vi "Phoenix.vi"(11 "Args":string[](array[string])) -> (2 "Logs":string, 3 "Exit":i32)   [LabVIEW 2020]
uses:
  Vision_class/Old vision/Controls/Estimadores.ctl
  Vision_class/Old vision/Decode SSL and Refree Wrapper Package Folder/SSL Referee Game Status.ctl
  Vision_class/Old vision/Draw Field Folder/DrawTargets.ctl
  Vision_class/Old vision/Controls/SSL Field State.ctl
  Vision_class/Old vision/Controls/SSL Detection Frame.ctl
  Vision_class/Old vision/Controls/SSL Detection Robot.ctl
  <vilib>/Analysis/Matrix/Datatypes/RealMatrix.ctl
  Vision_class/Old vision/Controls/SSL Detection Ball.ctl
  Communication_class/Communication.lvclass
  Controls/ComUDP.ctl
  Controls/ComSerial.ctl
  Controls/ComSOS.ctl
  Controls/vision_control.ctl
  Team_class/KeeperPlay.ctl
  Team_class/OffensivePlay.ctl
  Referee_class/command_interpreted.ctl
  Robot_class/roles.ctl
  Robot_class/tactics.ctl
  Team_class/DefensivePlay.ctl
  Parameters_class/Project.ctl
  Vision_class/Vision.lvclass
  Game_class/Game.lvclass
  Game_class/Game.lvclass/Game.ctl
  Parameters_class/Parameters.lvclass/Parameters.ctl
  Robot_class/Robot.lvclass
  Team_class/Team.lvclass/Team.ctl
  Events_class/Events.lvclass
  Referee_class/Referee.lvclass/Referee.ctl
  Robot_class/Robot.lvclass/Robot.ctl
  Game_class/Write Offensive ids.vi
  Game_class/Write Defensive ids.vi
  Game_class/Read Parameters.lvclass.vi
  Game_class/Write TestMode IDs.vi
  Game_class/Write TestMode.vi
  Game_class/Write Tests.vi
  Parameters_class/Write Area.vi
  Parameters_class/Write DistanceBehindAttacker.vi
  Parameters_class/Write DistanceInFrontOfAttacker.vi
  Parameters_class/Write DistanceStop.vi
  Parameters_class/Write DistanceToBallOut.vi
  Parameters_class/Write DistanceToGoAroundBall.vi
  Parameters_class/Write DistanceToGoAroundBallPass.vi
  Parameters_class/Write DistanceToKickingAngle.vi
  Parameters_class/Write Force++.vi
  Parameters_class/Write KickAngle.vi
  Parameters_class/Write KickEps.vi
  Parameters_class/Write KickForce.vi
  Parameters_class/Write KickRange.vi
  Parameters_class/Write MaxAcceleration.vi
  Parameters_class/Write MaxControlIncrement.vi
  Parameters_class/Write MaxDeceleration.vi
  Parameters_class/Write MaxOutputAngle.vi
  Parameters_class/Write MaxOutputXY.vi
  Parameters_class/Write MinDistToKick.vi
  Parameters_class/Write PassAngle.vi
  Parameters_class/Write Type of Marker.vi
  Parameters_class/Write AttackerFarback.vi
  Parameters_class/Write TouchDistance.vi
  Parameters_class/Write TimeoutDistanceInY.vi
  Parameters_class/Write TimeoutDistanceInX.vi
  Parameters_class/Write TimeoutDistanceBetweenRobots.vi
  Parameters_class/Write DistanceForPossession.vi
  Parameters_class/Write DistanceForaStillBall.vi
  Parameters_class/Write AngularToleranceForPossession.vi
  Parameters_class/Write AttakingOurselves.vi
  Parameters_class/Write Debug.vi
  Parameters_class/Write ChipKick activated.vi
  Parameters_class/Write Angle.vi
  Parameters_class/Write PID gains Vel.vi
  Parameters_class/Write PID gains Vel_desired.vi
  Parameters_class/Write PID gains Angle.vi
  Parameters_class/Write Number of Offesnive.vi
  Parameters_class/Write Shoot Out_.vi
  Parameters_class/Write DefenseAvoidArea.vi
  Parameters_class/Write InvertKick.vi
  Parameters_class/Write ShootOutForce.vi
  Parameters_class/Write dtPosEstBall.vi
  Parameters_class/Write SimplePass.vi
  Parameters_class/Write GoalieInFrontGoal.vi
  Parameters_class/Write RollToPass.vi
  Parameters_class/Write VelNearBall.vi
  Parameters_class/Write Project.vi
  Game_class/Write Parameters.lvclass.vi
  Game_class/Read DefensiveTeam.vi
  Game_class/Write DefensiveTeam.vi
  Team_class/Read RobotRef.vi
  Game_class/Read OffensiveTeam.vi
  Game_class/Read AllyRef.vi
  Game_class/Read KeeperTeam.vi
  Team_class/Write RobotRef.vi
  Game_class/Write NavigationTeam.vi
  Game_class/Write EventsRef.vi
  Game_class/Write OffensiveTeam.vi
  Game_class/Write KeeperTeam.vi
  Robot_class/Read id.vi
  Robot_class/Read role.vi
  Robot_class/Read tactic.vi
  Game_class/Read Referee.vi
  Team_class/Read DefensivePlay.vi
  Team_class/Read OffensivePlay.vi
  Team_class/Read KeeperPlay.vi
  Referee_class/Read command_interpreted.vi
  Ally_class/Ally.lvclass
  home/roboime/Documentos/VSS_AI/Team_class/Team.lvclass
  Parameters_class/Parameters.lvclass
  Playbook_class/Playbook.lvclass
  Referee_class/Referee.lvclass
  <vilib>/Analysis/Matrix/NI_Matrix.lvlib
panel:
  out "touch":bool
  in  "Debug":bool
  out "tempo udp":dbl
  in  "ball velocity máx":dbl=20.0
  in  "PID gains Angle":cluster{"(Kc)":dbl, "(Ki)":dbl, "(Kd)":dbl}={"(Kc)"=5.0, "(Ki)"=0.1, "(Kd)"=-1.0}
  in  "PID gains Vel D":cluster{"(Kp)":dbl, "(Ki)":dbl, "(Kd)":dbl}={"(Kp)"=20.0, "(Ki)"=100.0, "(Kd)"=0.5}
  in  "ChipKick activated":bool
  out "error out":errorcluster
  in  "Draw Graphs":bool
  out "zoom":dbl
  in  "Test":bool
  in  "Tab Control":T1(tab)
  in  "SEND?":bool=TRUE
  in  "VSSRef Replacement infos":T2={"Local IP:"="NADA", "Port"=10004, "Server IP:"="192.168.0.100"}
  in  "VSSRef":T3
  in  "Project":T4=enum."VSS"
  in  "Com UDP":T5={"UDP GrSim TX"=TRUE, "Address:"="172.31.17.157", "Port:"=20011}
  in  "Com Serial":T6={"Serial TX"=FALSE, "Porta:"="COM12"}
  in  "Com SOS":T7={"UDP SOS TX "=FALSE, "SOS Port: 2"=10025, "SOS Port: "=10021, "SOS Address:"="192.168.0.101"}
  in  "RefBox UDP RX":T2={"Local IP:"="", "Port"=10003, "Server IP:"="224.5.23.2"}
  out "RefBox RX":bool
  in  "Defense\n stretch":i32=2000
  in  "Defense\n width":i32=1000
  in  "Team":enum16{"Azul", "Amarelo"}(ring) caption="Enum"
  in  "Side":enum16{"Esquerdo", "Direito"}(ring) caption="Enum"
  in  "Goalie":string(combo)="0"
  in  "Command":string(combo)="Auto"
  in  "AttakingOurselves":bool
  out "SSL RX":bool
  in  "SSL UDP RX":T2={"Local IP:"="", "Port"=10002, "Server IP:"="224.0.0.1"}
  in  "FIRASim?":bool=TRUE
  out "KeeperPlay":T8=enum."NormalGame"
  out "OffensivePlay":T9=enum."TestPlay"
  out "Keeper Team":cluster{"id":i32, "role":T10, "tactic":T11}[](array[cluster])
  out "Offensive Team":cluster{"id":i32, "role":T10, "tactic":T11}[](array[cluster])
  out "Defensive Team":cluster{"id":i32, "role":T10, "tactic":T11}[](array[cluster])
  out "DefensivePlay":T12=enum."Halt"
  in  "TestMode IDS":dbl[](array[numeric])
  out "SSL Referee Game Status":T13 {"Time" format="%<%.3X %x>T"; "Blue Timeout Remaining" format="%<%M:%S>t"; "Yellow Timeout Remaining" format="%<%M:%S>t"; "Time Left" format="%<%M:%S>t"}
  out "FPS Offensive":dbl
  out "FPS SetParameters":dbl
  out "FPS Defensive":dbl
  out "FPS Keeper":dbl
  out "FPS Com":dbl
  out "FPS Draw Field":dbl
  out "FPS Graph":dbl
  out "FPS referee":dbl
  out "FPS vision":dbl
  out "FPS Events":dbl
  out "FPS Mouse":dbl
  out "FPS Print Field":dbl
  in  "zigzag Points":cluster{"x":dbl, "y":dbl, "Angle":dbl}[](array[cluster])=[{"x"=-4300.0, "y"=-3000.0, "Angle"=0.0}, {"x"=-4300.0, "y"=3000.0, "Angle"=0.0}, {"x"=-100.0, "y"=3000.0, "Angle"=0.0}, {"x"=-4300.0, "y"=3000.0, "Angle"=0.0}]
  in  "TestMode":bool
  in  "Tests":enum16{"zigzag", "goto"}(ring)
  in  "Offensive ids":dbl[](array[numeric])
  in  "Defensive ids":dbl[](array[numeric])
  out "command_interpreted":T14=enum."Halt"
  out "FPS Navigation":dbl
  out "FPS Read UDP":dbl
  in  "id 3":dbl
  in  "id 2":dbl
  in  "id 1":dbl
  out "Robot":cluster{"Modulo":dbl, "Modulo":dbl}(graph)
  out "Robot":cluster{"Modulo":dbl, "Modulo":dbl}(graph)
  out "Robot":cluster{"Modulo":dbl, "Modulo":dbl}(graph)
  out "ball":dbl(graph)
  in  "Tab Control 2":enum32{"SSL Params", "VSS Params"}(tab)
  in  "AI Parameters":T15={"Defensive Marker"=enum."SecondMostDangerous", "TimeoutDistanceInX"=600.0, "TimeoutDistanceInY"=600.0, "DistanceForStealBall"=0.0, "TouchDist"=130.0, "AttackerFarback"=1500.0, "MinDistToKick"=150.0, "Type of Marker"=enum."BlockEnemyPass", "Type of Defense "=enum."Manmark", "PassAngle"=0.045, "KickRange"=60.0, "KickForce"=100.0, "KickEps"=0.05, "KickAngle"=0.09, "Force++"=15.0, "DistanceToKickingAngle"=150.0, "DistanceToBallOut"=600.0, "DistanceStop"=600.0, "DistanceBehindAttacker"=200.0, "Area"=enum."Square", "DistForPossession"=180.0, "DistanceToGoAroundBallPass"=0.0, "DistanceToGoAroundBall"=200.0, "DistanceInFrontOfAttacker"=200.0, "TimeoutDistanceBetweenRobots"=300.0, "MaxOutputAngle"=4.0, "MaxOutputXY"=1.8, "MaxDeceleration"=1.0, "MaxControlIncrement"=1.0, "MaxAcceleration"=4.0, "AngularToleranceForPossession"=0.3, "MaxVelBallToBeginDuelist"=0.5, "ZigZagAngle"=0.0, "PID gains Vel"={"(Kc)"=0.0, "(Ti, min)"=0.0, "(Td, min)"=0.0}, "Number of Offensive"=enum."Auto", "Shoot Out?"=FALSE, "DefenseAvoidArea"=FALSE, "InvertKick"=[], "shootOutForce "=5.0, "dtPosEst\nBall"=0.3, "AttackerIgnoreBallObstacle"=500.0, "BarrierDistanceToArea"=150.0, "SimplePass"=FALSE, "GoalieInFront\nGoal"=90.0, "RollToPass"=FALSE, "VelNearBall"=0.3, "OldRRT"=FALSE}
  in  "AI Parameters VSS":T16={"Robots ids"={"Goalie"=enum."0", "Attacker"=enum."1", "Defender"=enum."2"}}
  in  "Id camera\ninf dir":dbl=2.0
  in  "Id camera\ninf esq":dbl
  in  "Id camera\nsup dir":dbl=3.0
  in  "Id camera\nsup esq":dbl=1.0
  in  "ignore left?":bool
  in  "ignore rigth?":bool
  in  "Estimador":T17
  in  "Draw Targets?":T18={"Attacker"=TRUE, "Striker"=TRUE, "Goalie"=TRUE, "Defender"=TRUE, "kick"=TRUE, "Est Ball"=TRUE, "Est Robot"=FALSE, "Path S"=FALSE, "Path C"=FALSE, "Dngr.Enemy"=TRUE, "2nd Striker"=TRUE}
  in  "Draw Field":bool=TRUE
  in  "Communication in":refnum<class "Communication.lvclass">
  in  "Frame and Field Size out Ref":T19 {"Detection Frame Out"."robots_blue"."height" format="%+4.3f"; "Detection Frame Out"."robots_blue"."pixel_y" format="%+4.3f"; "Detection Frame Out"."robots_blue"."pixel_x" format="%+4.3f"; "Detection Frame Out"."robots_blue"."orientation" format="%+4.3f"; "Detection Frame Out"."robots_blue"."y" format="%+4.3f"; "Detection Frame Out"."robots_blue"."confidence" format="%4.3f"; "Detection Frame Out"."robots_blue"."x" format="%+4.3f"; "Detection Frame Out"."robots_yellow"."height" format="%+4.3f"; "Detection Frame Out"."robots_yellow"."pixel_y" format="%+4.3f"; "Detection Frame Out"."robots_yellow"."pixel_x" format="%+4.3f"; "Detection Frame Out"."robots_yellow"."orientation" format="%+4.3f"; "Detection Frame Out"."robots_yellow"."y" format="%+4.3f"; "Detection Frame Out"."robots_yellow"."confidence" format="%4.3f"; "Detection Frame Out"."robots_yellow"."x" format="%+4.3f"}
  out "2D Picture":picture
  in  "SSL Referee Game Status Ref":T13 {"Time" format="%<%.3X %x>T"; "Blue Timeout Remaining" format="%<%M:%S>t"; "Yellow Timeout Remaining" format="%<%M:%S>t"; "Time Left" format="%<%M:%S>t"}
  out "GUI Game Status":T13 {"Time" format="%<%.3X %x>T"; "Blue Timeout Remaining" format="%<%M:%S>t"; "Yellow Timeout Remaining" format="%<%M:%S>t"; "Time Left" format="%<%M:%S>t"}
  # "To execute Test and TestMode(zigzag)\nthe referee command must be Stop"
  # "PID gains vel:\nmakes the estimated velocity\ngoes closer into the desired velocity"
  # "Score"
  # "Red Cards"
  # "Yellow Cards"
  # "Timeouts Left"
  # "Timeout Remaining"
  # "Goalie ID"
  # "left goal"
  # "right goal"
  # "vision computer"
  # "Score"
  # "Red Cards"
  # "Yellow Cards"
  # "Timeouts Left"
  # "Timeout Remaining"
  # "Goalie ID"
  # "Score"
  # "Red Cards"
  # "Yellow Cards"
  # "Timeouts Left"
  # "Timeout Remaining"
  # "Goalie ID"
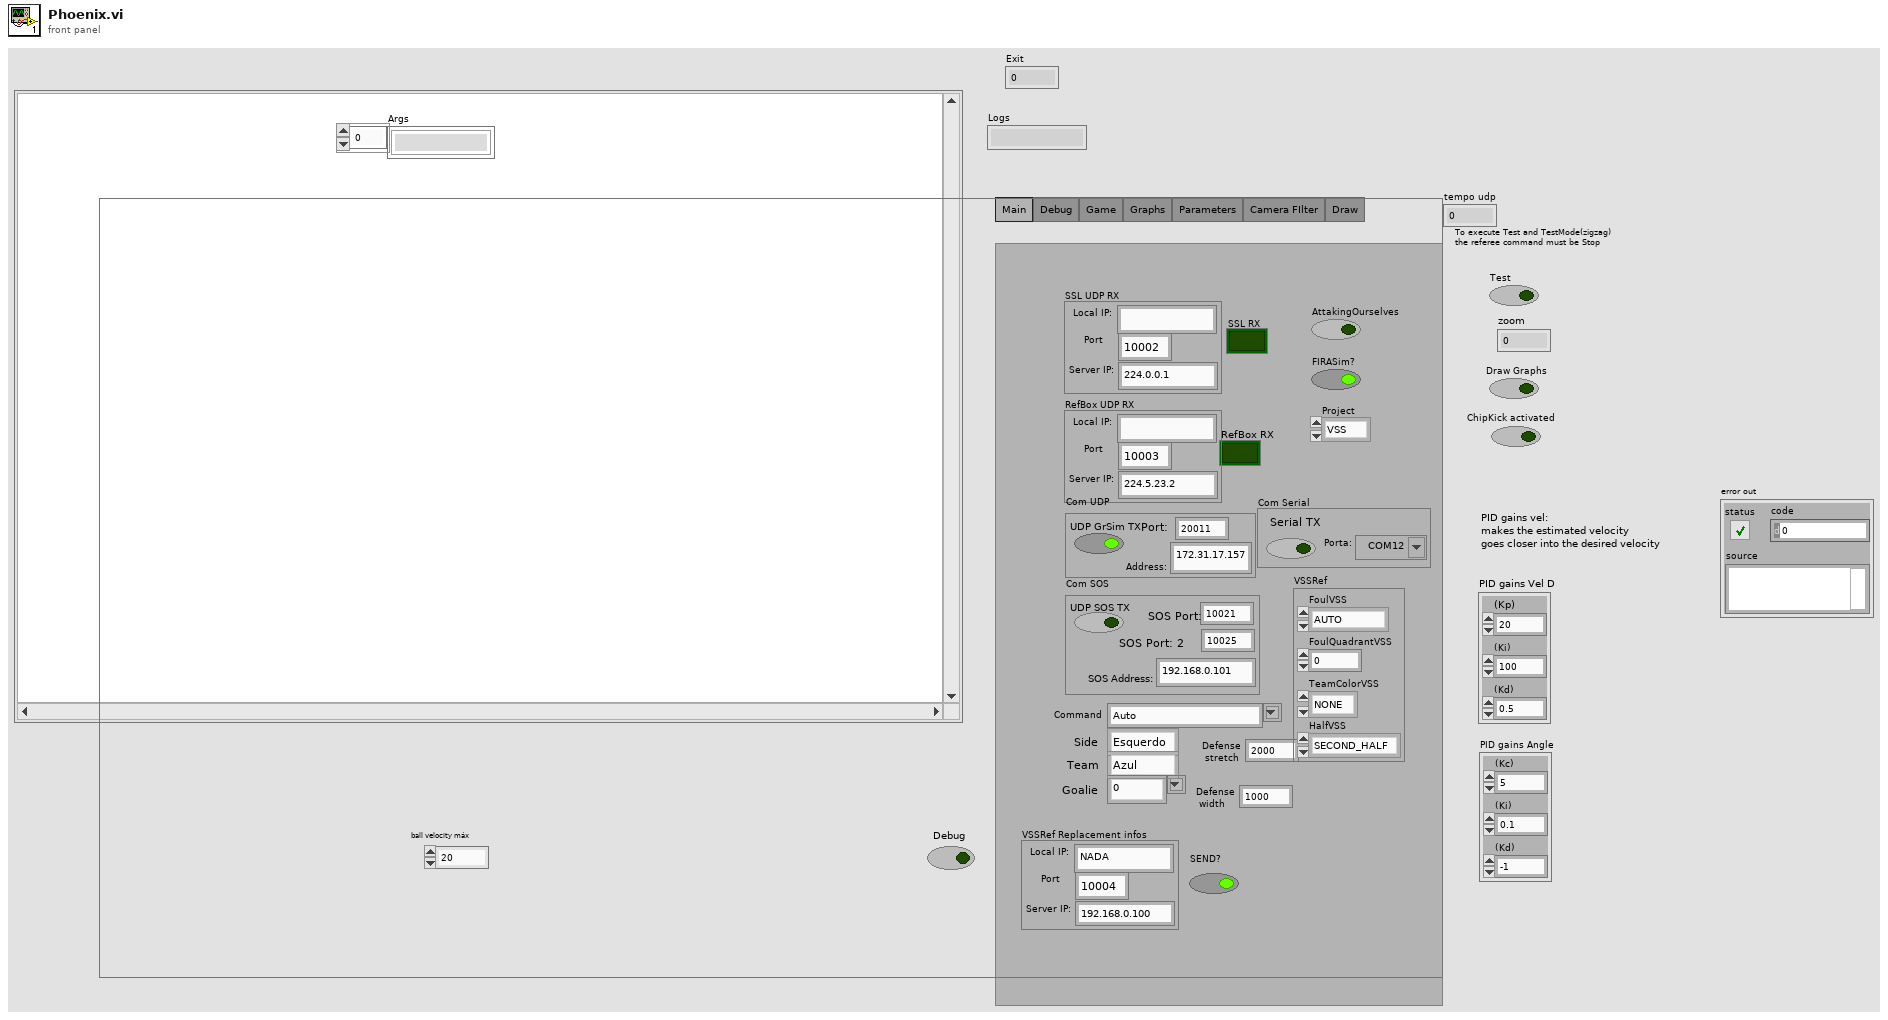
[diagram p1: front panel]
types:
  T1 = enum32{"Main", "Debug", "Game", "Graphs", "Parameters", "Camera FIlter", "Draw"}
  T2 = typedef "vision_control.ctl" = cluster{"Local IP:":string, "Port":i32, "Server IP:":string}
  T3 = cluster{"FoulVSS":enum16{"AUTO", "GAME_ON", "STOP", "KICKOFF", "FREE_BALL", "GOAL_KICK", "PENALTY_KICK", "FREE_KICK"}, "FoulQuadrantVSS":dbl, "TeamColorVSS":enum16{"NONE", "YELLOW", "BLUE"}, "HalfVSS":enum16{"SECOND_HALF", "FIRST_HALF", "NO_HALF"}}
  T4 = typedef "Project.ctl" = enum16{"SSL", "VSS"}
  T5 = typedef "ComUDP.ctl" = cluster{"UDP GrSim TX":bool, "Address:":string, "Port:":u16}
  T6 = typedef "ComSerial.ctl" = cluster{"Serial TX":bool, "Porta:":refnum<visa-resource-name>}
  T7 = typedef "ComSOS.ctl" = cluster{"UDP SOS TX ":bool, "SOS Port: 2":u16, "SOS Port: ":u16, "SOS Address:":string}
  T8 = typedef "KeeperPlay.ctl" = enum16{"ZigZag", "Goto", "NormalGame", "KeeperPlay", "Halt", "Timeout", "PenaltyEnemy", "TestPlay"}
  T9 = typedef "OffensivePlay.ctl" = enum16{"TableWithStriker", "TableWith2ndStrikerPlay", "PrepareDoublePass", "PrepareRollToPass", "SimplePass", "PreparePass", "PassToStriker", "BallOutOfField", "PassTo2ndStriker", "StopOffensive", "Prepare Penalty Enemy", "EnemyPossessionAtEnemyField", "EnemyPossesionAtOurField", "TestPlay", "PreparePenaltyAlly", "KickPenaltyAlly", "PrepareKickoffAlly", "PrepareKickoffEnemy", "IndirectEnemy", "DirectEnemy", "NormalGame", "DirectKick", "Pass", "Halt", "Timeout", "PassPlay", "PenaltyEnemy"}
  T10 = typedef "roles.ctl" = enum16{"BallChallengerAttackerVSS", "NormalAttackerVSS", "AttackerAimGoalVSS", "DefenderAreaVSS", "KeeperVSS", "Tabler", "TableFinalizer", "PrepareRollToPassRoller", "PrepareRollToPassReceiver", "SimplePassRoll", "SimplePassRollReceiver", "PenaltyDefense", "PreparePassReceiver 2", "PreparePassReceiver 1", "PassObserver", "Timeout", "Goto", "ZigZag", "None", "BallOutOfField", "DefenderArea", "Duelist", "AttackerStop", "FollowAttacker", "KeeperRole", "KickPenalty", "AttackerAimGoal", "AttackerBlock", "Marker", "Halt", "Shoot", "PassKicker", "PassReceiver", "TestRole", "PenaltyAttacker"}
  T11 = typedef "tactics.ctl" = enum16{"ReceivePassInFuturePoint", "Roller", "PrepareRollToPassRollerGoTo", "PrepareRollToPassReceiverGoTo", "WaitRoll", "PositionToRoll", "PenaltyAttacker", "PassObserver", "PenaltyDefense", "TableReceiverTactic", "Test", "DefendGoal", "Marker", "FollowAttacker", "DefendArea", "Shoot", "AttackerAimGoal", "AttackerBallOutOfField", "AttackerBlock", "AttackerStop", "Duelist", "Halt", "ZigZag", "GoTo", "Timeout", "KickToPassReceiver", "PositionToReceivePass", "DefendAreaVSS", "DefendGoalVSS", "KickVSS", "AttackVSS", "DispBallVSS", "PenaltyAttackVSS", "WaitPass"}
  T12 = typedef "DefensivePlay.ctl" = enum16{"NormalDefensiveWithDuelist", "NormalDefensive", "TestPlay", "Halt", "Timeout", "PenaltyEnemy", "PenaltyAlly"}
  T13 = typedef "SSL Referee Game Status.ctl" = cluster{"Stage":string, "Command":string, "Time Left":dbl, "Yellow Team":string, "Blue Team":string, "Yellow Score":u32, "Blue Score":u32, "Yellow Red Cards":u32, "Blue Red Cards":u32, "Yellow Yellow Cards":u32, "Blue Yellow Cards":u32, "Yellow Timeouts Left":u32, "Blue Timeouts Left":u32, "Yellow Timeout Remaining":dbl, "Blue Timeout Remaining":dbl, "Yellow Goalie Id":u32, "Blue Goalie Id":u32, "Time":timestamp}
  T14 = typedef "command_interpreted.ctl" = enum16{"Goal Ally", "Goal Enemy", "Ball Placement Enemy", "Ball Placement Ally", "Normal Half Time", "Extra Time  Break", "Extra Half Time", "None", "Post Game", "PKA Normal Start", "Prepare Kickoff Ally", "PKE Normal Start", "Prepare Kickoff Enemy", "Force Start", "Halt", "Timeout", "Prepare Penalty Ally", "Prepare Penalty Enemy", "PPA NormalStart", "PPE Normal Start", "Indirect Free Ally", "Direct Free Enemy", "Direct Free Ally", "Indirect Free Enemy", "Stop"}
  T15 = cluster{"Defensive Marker":enum16{"SecondMostDangerous", "MostDangerous"}, "TimeoutDistanceInX":dbl, "TimeoutDistanceInY":dbl, "DistanceForStealBall":dbl, "TouchDist":dbl, "AttackerFarback":dbl, "MinDistToKick":dbl, "Type of Marker":enum16{"BlockEnemyPass", "BlockOurGoal"}, "Type of Defense ":enum16{"Barreira", "Manmark"}, "PassAngle":dbl, "KickRange":dbl, "KickForce":dbl, "KickEps":dbl, "KickAngle":dbl, "Force++":dbl, "DistanceToKickingAngle":dbl, "DistanceToBallOut":dbl, "DistanceStop":dbl, "DistanceBehindAttacker":dbl, "Area":enum16{"Circular", "Square"}, "DistForPossession":dbl, "DistanceToGoAroundBallPass":dbl, "DistanceToGoAroundBall":dbl, "DistanceInFrontOfAttacker":dbl, "TimeoutDistanceBetweenRobots":dbl, "MaxOutputAngle":dbl, "MaxOutputXY":dbl, "MaxDeceleration":dbl, "MaxControlIncrement":dbl, "MaxAcceleration":dbl, "AngularToleranceForPossession":dbl, "MaxVelBallToBeginDuelist":dbl, "ZigZagAngle":dbl, "PID gains Vel":cluster{"(Kc)":dbl, "(Ti, min)":dbl, "(Td, min)":dbl}, "Number of Offensive":enum16{"6", "5", "4", "3", "2", "1", "0", "Auto"}, "Shoot Out?":bool, "DefenseAvoidArea":bool, "InvertKick":dbl[], "shootOutForce ":dbl, "dtPosEst\nBall":dbl, "AttackerIgnoreBallObstacle":dbl, "BarrierDistanceToArea":dbl, "SimplePass":bool, "GoalieInFront\nGoal":dbl, "RollToPass":bool, "VelNearBall":dbl, "OldRRT":bool}
  T16 = cluster{"Robots ids":cluster{"Goalie":enum16{"auto", "5", "4", "3", "2", "1", "0"}, "Attacker":enum16{"auto", "5", "4", "3", "2", "1", "0"}, "Defender":enum16{"auto", "5", "4", "3", "2", "1", "0"}}}
  T17 = typedef "Estimadores.ctl" = enum16{"4thDerivate", "2ndDerivate", "Nenhum", "Simples", "Kalman"}
  T18 = typedef "DrawTargets.ctl" = cluster{"Attacker":bool, "Striker":bool, "Goalie":bool, "Defender":bool, "kick":bool, "Est Ball":bool, "Est Robot":bool, "Path S":bool, "Path C":bool, "Dngr.Enemy":bool, "2nd Striker":bool}
  T19 = typedef "SSL Field State.ctl" = cluster{"Detection Frame Out":T20, "Field Size Out":cluster{"line_width":u32, "field_length":u32, "field_width":u32, "boundary_width":u32, "referee_width":u32, "goal_width":u32, "goal_depth":u32, "goal_wall_width":u32, "center_circle_radius":u32, "defense_radius":u32, "defense_stretch":u32, "free_kick_from_defense_dist":u32, "penalty_spot_from_field_line_dist":u32, "penalty_line_from_spot_dist":u32}, "Received Time Stamp":timestamp}
  T20 = typedef "SSL Detection Frame.ctl" = cluster{"frame_number":u32, "t_capture":dbl, "t_sent":dbl, "camera_id":u32, "robots_yellow":T21[], "robots_blue":T21[], "balls":T23[], "Valid":bool, "Time Stamp":timestamp, "New":bool, "Initialized":bool}
  T21 = typedef "SSL Detection Robot.ctl" = cluster{"x":sgl, "robot_id":u32, "confidence":sgl, "y":sgl, "orientation":sgl, "pixel_x":sgl, "pixel_y":sgl, "height":sgl, "Valid":bool, "Time Stamp":timestamp, "x_k|k":T22, "Pk|k":T22, "Previous Time Stamp":timestamp, "R":T22, "vx":dbl, "vy":dbl, "vang":dbl}
  T22 = typedef "NI_Matrix.lvlib/RealMatrix.ctl" = dbl[][]
  T23 = typedef "SSL Detection Ball.ctl" = cluster{"x":sgl, "area":u32, "confidence":sgl, "y":sgl, "z":sgl, "pixel_x":sgl, "pixel_y":sgl, "Valid":bool, "Time Stamp":timestamp, "x_k|k":T22, "Pk|k":T22, "Id":u32, "Previous Time Stamp":timestamp, "R":T22, " vx":sgl, "vy":dbl, "vz":dbl}
  T24 = typedef "AI Input.ctl" = cluster{"our_robots":T25[], "enemy_robots":T25[], "balls":T31[], "geometry":T32, "IA Judge":T33, "Received Timestamp":timestamp, "Events":T35}
  T25 = typedef "AI Robot.ctl" = cluster{"id":u32, "function":T26, "x":dbl, "y":dbl, "orientation":dbl, "v_tangent":dbl, "v_normal":dbl, "v_ang":dbl, "kick_x":dbl, "kick_z":dbl, "dribble":bool, "Timestamp":timestamp, "estimatives":cluster{"est_v_tangent":dbl, "est_v_normal":dbl, "est_vx":dbl, "est_vy":dbl, "Pos Robot Est":dbl[]}, "dest_x_kick":dbl, "dest_y_kick":dbl, "Gap Coord":dbl[], "States":T27, "Path ":dbl[][], "Path  Smooth":dbl[][], "Dest":T28, "vx_desired":dbl, "vy_desired":dbl, "slowBehavior":bool, "VSSStates":T30}
  T26 = typedef "Functions Enum.ctl" = enum16{"2nd Striker", "Attacker", "Goalie", "Defender", "Striker", "Goto 0", "Dummy", "Kicker", "ZigZag 0", "ZigZag 1", "ZigZag 2", "ZigZag 3", "ZigZag 4", "ZigZag 5", "ZigZag 6", "ZigZag 7", "ZigZag 8", ""}
  T27 = typedef "AttackerStates.ctl" = enum16{"Pass", "GoToTangent", "BallGetting", "GoToKick", ""}
  T28 = typedef "PathDests.ctl" = T29[]
  T29 = typedef "PathDest.ctl" = cluster{"dest_x":dbl, "dest_y":dbl, "dest_orientation":dbl, "dest_vel":dbl}
  T30 = typedef "VSSAttackerStates.ctl" = enum16{"Pass", "GoToTangent", "BallGetting", "GoToKick", "Rotate anti-clockwise", "Rotate Clockwise", ""}
  T31 = typedef "AI Ball.ctl" = cluster{"x":dbl, "y":dbl, "timestamp":timestamp, "Vel_x":dbl, "Vel_y":dbl, "Pos Bola Est":dbl[], "Valid":bool}
  T32 = typedef "Field Size.ctl" = cluster{"line_width":u32, "field_length":u32, "field_width":u32, "boundary_width":u32, "referee_width":u32, "goal_width":u32, "goal_depth":u32, "goal_wall_width":u32, "center_circle_radius":u32, "defense_radius":u32, "defense_stretch":u32, "free_kick_from_defense_dist":u32, "penalty_spot_from_field_line_dist":u32, "penalty_line_from_spot_dist":u32}
  T33 = typedef "AI Judge.ctl" = cluster{"stage":string, "command":string, "our_goalie_id":dbl, "enemy_goalie_id":dbl, "command enum":T34, "Time":enum16{"Azul", "Amarelo"}}
  T34 = typedef "Command Enum.ctl" = enum16{"Halt", "Stop", "Force Start", "PKA Normal Start", "Prepare Kickoff Ally", "PKE Normal Start", "Prepare Kickoff Enemy", "Prepare Penalty Ally", "PPA Normal Start", "Prepare Penalty Enemy", "PPE Normal Start", "Direct Free Enemy", "Direct Free Ally", "Indirect Free Enemy", "Indirect Free Ally", "Timeout Enemy", "Timeout Ally", "Goal Enemy", "Goal Ally", "Ball Placement Enemy", "Ball Placement Ally", "Normal Half Time", "Extra Time Break", "Extra Half Time", "None", "Post Game"}
  T35 = typedef "Events.ctl" = cluster{"Touch":bool, "Ball out":bool, "id touch":dbl, "Ball out of \nVision":bool, "Ball inside \nGoalie area":bool, "Robot not responding":bool, "Robots responding status":dbl[], "Enemy Ball \nPossession":bool, "Pass State":bool, "id end of pass":dbl, "Kick":bool, "Id ini Possession":dbl, "Ball Possesion":bool, "Id Possesion":dbl, "Direct Kick":bool, "2nd Strk Ativo":bool}
  T36 = cluster{"Varint":u32, "Varint":u32, "Varint":u32, "Double":dbl, "Varint":u32}
  T37 = enum16{"FreeBall", "PrepareFreeBall", "GoalKickEnemy", "GoalKickAlly", "KickoffAlly", "KickoffEnemy", "PrepareGoalKickEnemy", "PrepareGoalKickAlly", "Stop", "PrepareKickoffEnemy", "PrepareKickoffAlly", "PreparePenaltyEnemy", "Timeout", "DeadBall", "NormalGame", "KickPenaltyAlly", "PenaltyEnemy", "BallChallenge", "PreparePenaltyAlly", "Halt"}
  T38 = enum16{"FreeBall", "PrepareFreeBall", "GoalKickEnemy", "GoalKickAlly", "KickoffAlly", "KickoffEnemy", "PrepareGoalKickEnemy", "PrepareGoalKickAlly", "Stop", "PrepareKickoffEnemy", "PrepareKickoffAlly", "PreparePenaltyEnemy", "Timeout", "DeadBall", "NormalGame", "KickPenaltyAlly", "PenaltyEnemy", "BallChallenge", "PreparePenaltyAlly", "Halt"}[]
  T39 = cluster{"(Kc)":dbl, "(Ti, min)":dbl, "(Td, min)":dbl}
  T40 = enum16{"6", "5", "4", "3", "2", "1", "0", "Auto"}
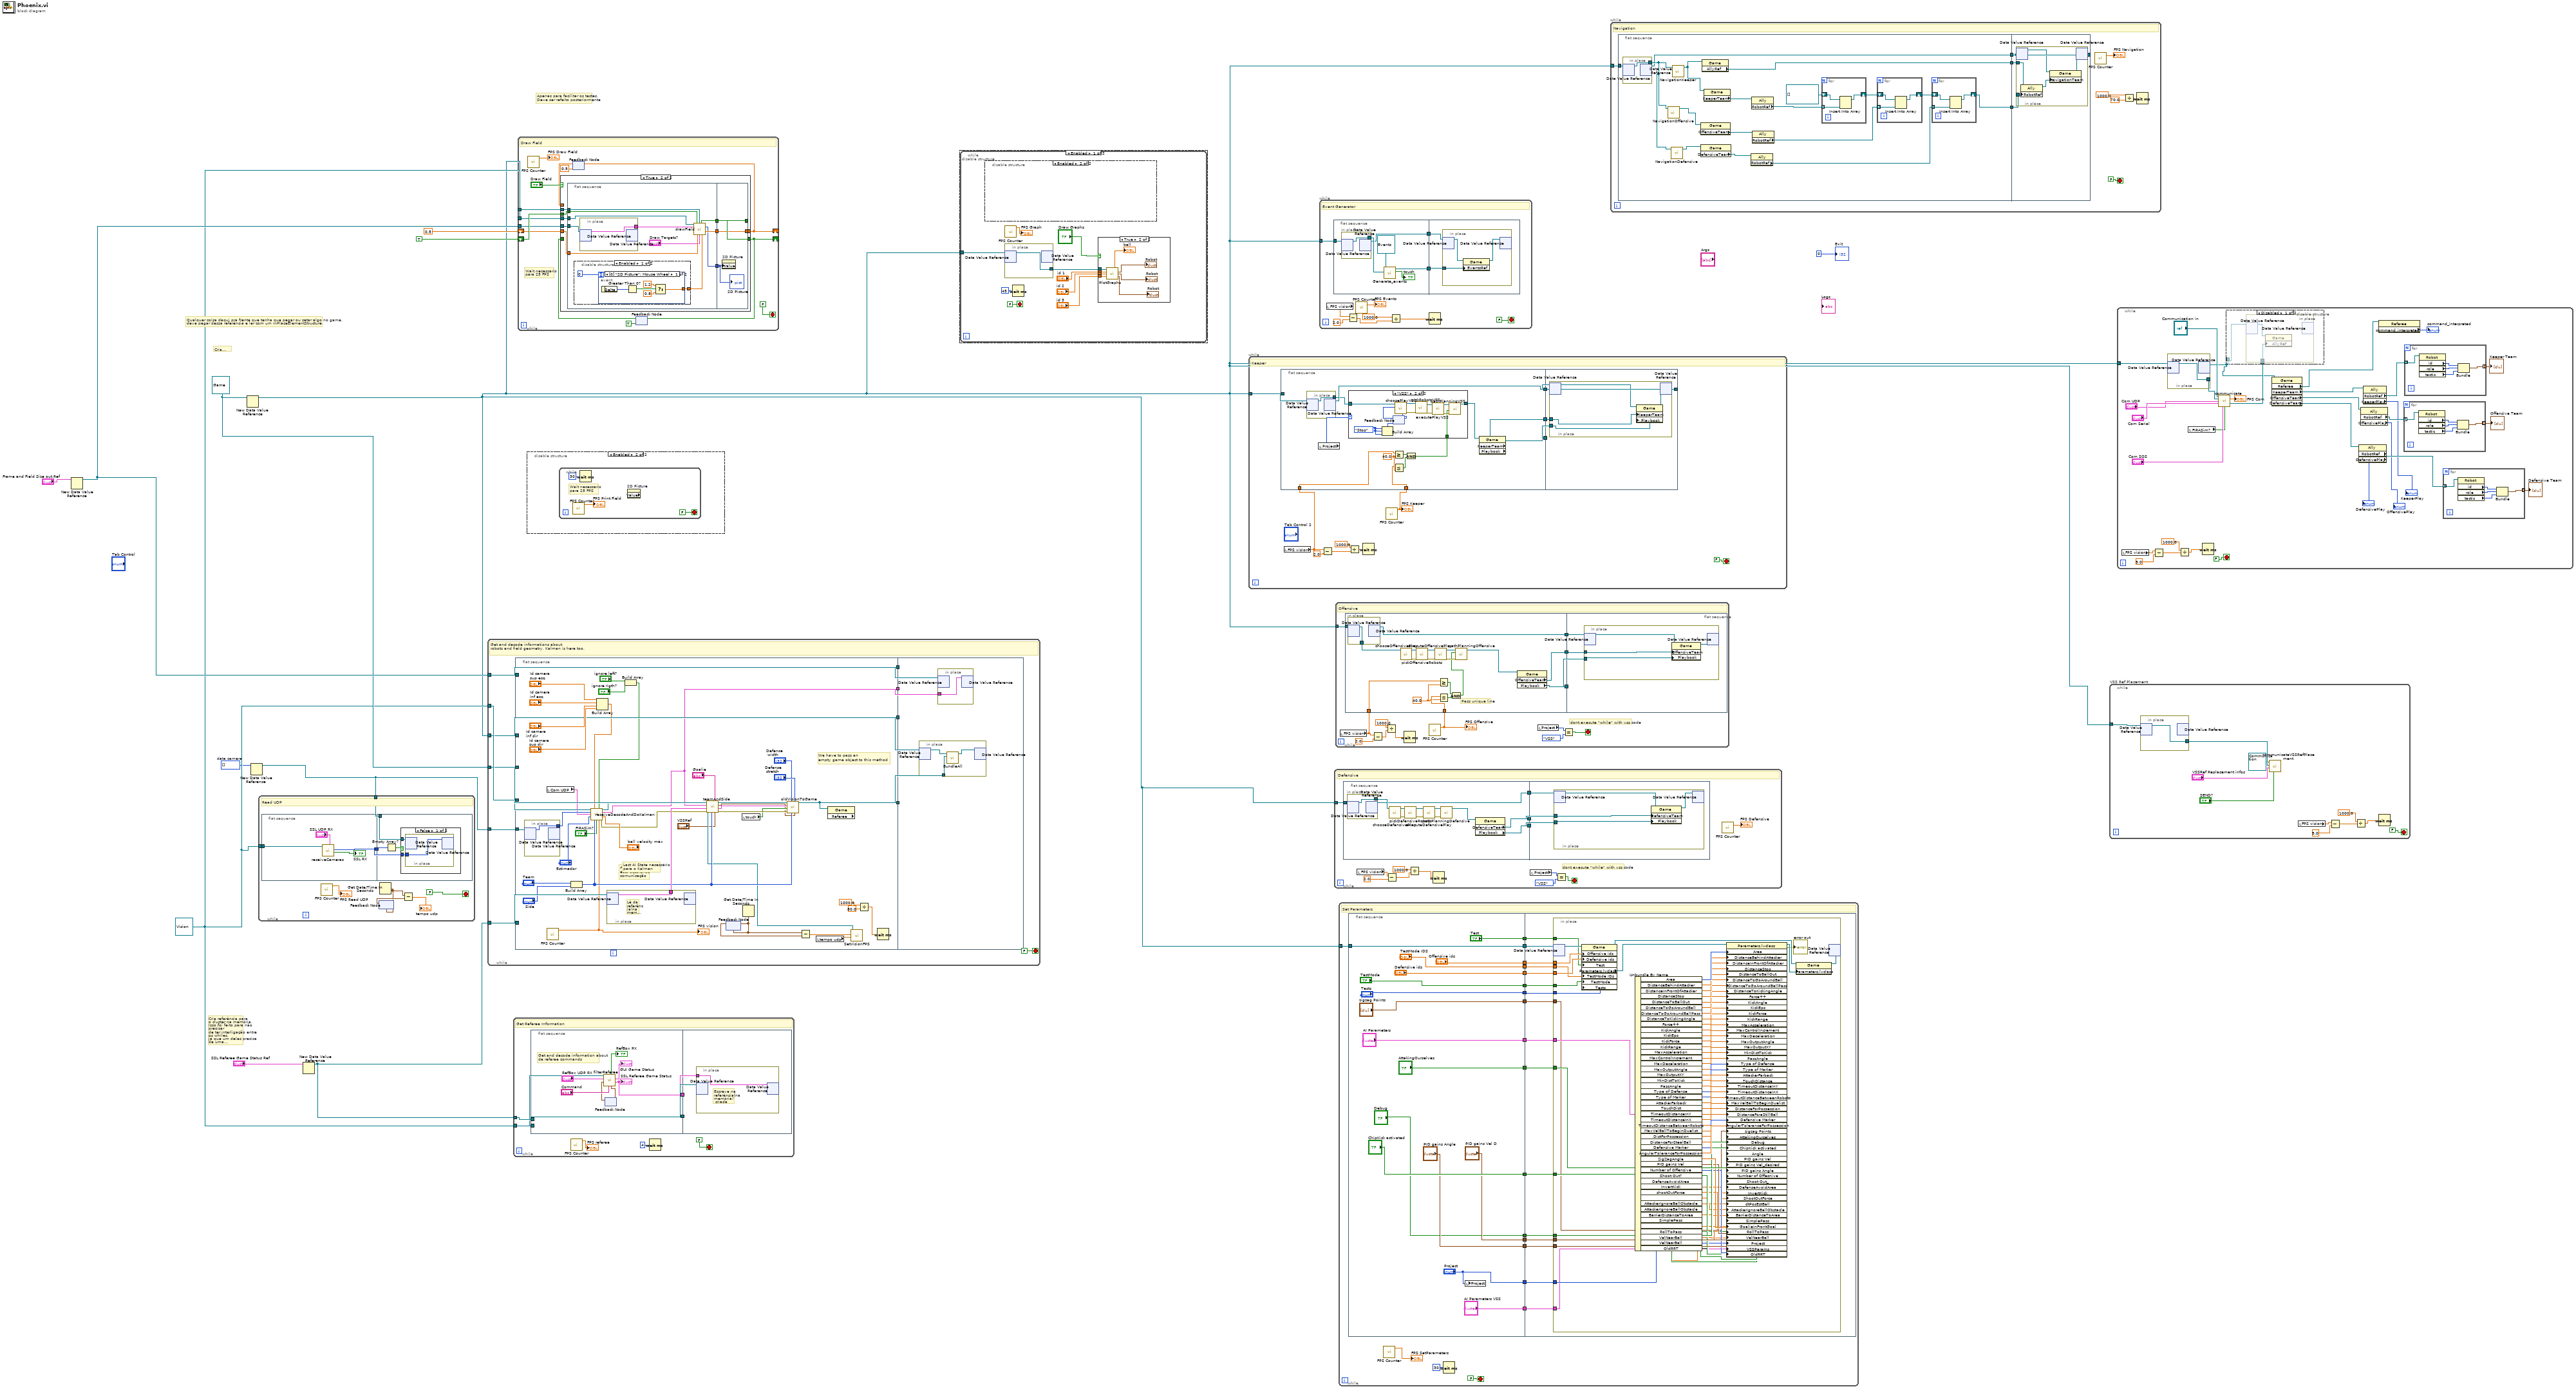
[diagram p0: block diagram]
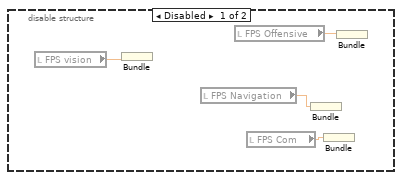
[diagram p3: hidden frame]
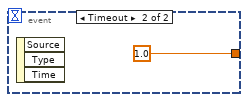
[diagram p7: hidden frame]
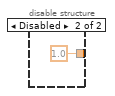
[diagram p8: hidden frame]
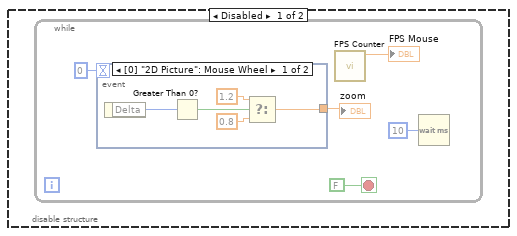
[diagram p9: hidden frame]
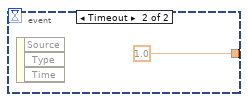
[diagram p10: hidden frame]
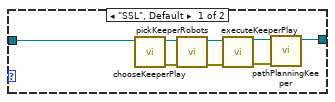
[diagram p11: hidden frame]
diagram:
  w4 = u8[] []  # data camera
  w6 = refnum<class "Game.lvclass"> refnum ("Game")
  w5 = refnum<class "Vision.lvclass"> refnum ("Vision")
  # "Apenas para facilitar os testes.\nDeve ser refeito posteriormente"
  # "Qualquer coisa daqui pra frente que tenha que pegar ou setar algo no game,\ndeve pegar dessa referência e ler com um InPlaceElementStructure"
  # "Cria referência pro game"
  # "Cria referência para\no cluster na memória.\nIsso foi feito para não precisar\nde ter interligação entre os whiles,\njá que um deles precisa de uma\nsaída do outro."
  n1 = New Data Value Reference(data value="Frame and Field Size out Ref") -> (data value reference=w7:refnum<data-value>)  [unwired: 1 in, 1 out]
  n2 = New Data Value Reference(data value=w6) -> (data value reference=w2:refnum<data-value>)  [unwired: 1 in, 1 out]
  n3 = New Data Value Reference(data value=w4) -> (data value reference=w3:refnum<data-value>)  [unwired: 1 in, 1 out]
  n4 = while {
    tunnel: w5 -> [w19]
    tunnel: w3 -> [w18]
    stop <- FALSE stop-if-true
    # "Read UDP"
    n5 = flat-sequence {
      tunnel: w19 -> [w23]
      tunnel: [w22] -> w17
      tunnel: w18 -> [w27]
      tunnel: w17 -> [w26]
      frame #0 {
        n6 = call "receiveCameras.vi"("Cluster"="SSL UDP RX", "Vision in"=w23) -> ("RX"=→"SSL RX":bool, "data camera out"=w22:u8[])  [unwired: 5 in, 2 out]
      }
      frame #1 {
        n7 = Empty Array?(array=w26) -> (empty?=w25:bool)
        n8 = case shown="False" w25 {
          tunnel: w27 -> [w29 _]
          tunnel: w26 -> [w28 _]
          frame False {
            n9 = in-place {
              in-place-border: w28 -> [w30]
              n10 = in-place-dvr #1(w29) -> ()  [unwired: 2 out]
              n11 = in-place-dvr #1(w30) -> ()  [unwired: 2 out]
            }
          }
          frame True {
          }
        }
      }
    }
    n12 = call "FPS Counter.vi"() -> ("Numeric"=→"FPS Read UDP":dbl)  [unwired: 11 in]
    n13 = Get Date/Time In Seconds() -> (seconds since 1Jan1904=w14:timestamp)
    n14 = feedback #2(w14) -> (w15:timestamp)
    n15 = feedback-in #2(w14) -> ()
    n16 = Subtract(x=w14, y=w15) -> (x-y=→"tempo udp":dbl)
  }
  n17 = New Data Value Reference(data value="SSL Referee Game Status Ref") -> (data value reference=w11:refnum<data-value>)  [unwired: 1 in, 1 out]
  n18 = while {
    tunnel: w5 -> [w40]
    tunnel: w11 -> [w39]
    tunnel: w2 -> [w36]
    tunnel: w7 -> [w37]
    tunnel: w6 -> [w38]
    tunnel: w3 -> [w31]
    stop <- FALSE stop-if-true
    # "Get and decode informations about\nrobots and field geometry. Kalman is here too."
    n19 = flat-sequence {
      tunnel: w40 -> [w62]
      tunnel: w39 -> [w83]
      tunnel: w38 -> [w69]
      tunnel: w37 -> [w71]
      tunnel: w36 -> [w70]
      tunnel: [w44] -> w35
      tunnel: [w60] -> w34
      tunnel: [w71] -> w33
      tunnel: [w70] -> w32
      tunnel: w31 -> [w67]
      tunnel: w35 -> [w89]
      tunnel: w34 -> [w87]
      tunnel: w33 -> [w88]
      tunnel: w32 -> [w90]
      frame #0 {
        # "We have to pass an\nempty game object to this method"
        # "Acende quando\nestá occorendo\ncomunicação"
        # "Last AI State necessário\npara o Kalman"
        n20 = in-place {
          in-place-border: [w85] -> w63
          n21 = in-place-dvr #3(w67) -> (w85:u8[])  [unwired: 1 out]
          n22 = in-place-dvr #3() -> ()  [unwired: 1 in, 2 out]
        }
        n23 = local read "Com UDP"() -> (w57:T5)
        n24 = call "FPS Counter.vi"() -> ("Numeric"=w54:dbl)  [unwired: 11 in]
        "FPS vision" <- w54
        n25 = Build Array("Team", "Side") -> (w59:u16[])
        n26 = Build Array("Id camera\nsup esq", "Id camera\ninf esq", "Id camera\ninf dir", "Id camera\nsup dir") -> (w64:dbl[])
        n27 = in-place {
          in-place-border: [w86] -> w84
          # "Lê da\nreferência(na memória)\ncriada"
          n28 = in-place-dvr #4(w83) -> (w86:T13)  [unwired: 1 out]
          n29 = in-place-dvr #4() -> ()  [unwired: 1 in, 2 out]
        }
        n30 = Build Array("ignore left?", "ignore rigth?") -> (w61:bool[])
        n31 = call "receiveDecodeAndDoKalman.vi"("Vision in"=w62, "cameras array"=w64, "Ignore left/rigth?"=w61, "unsigned byte array"=w63, "Com UDP"=w57, "Estimador"="Estimador", "max ball vel"="ball velocity máx", "team/side"=w59, "FIRASim?"="FIRASim?", "Fps"=w54) -> ("Vision out"=w55:refnum<class "Vision.lvclass">, "Frame and Field Size out"=w60:T19, "error out"=w58:errorcluster)  [unwired: 3 in]
        n32 = call "teamAndSide.vi"("VSSRef"="VSSRef", "Goalie"="Goalie", "team/side"=w59, "error in (no error)"=w58, "Game Status"=w84, "Field State Input"=w60, "Vision in"=w55) -> ("error out"=w80:errorcluster, "IA State"=w56:T24, "VSSRefOut"=w42:T3)  [unwired: 1 in, 1 out]
        n33 = local read "touch"() -> (w49:bool)
        n34 = Get Date/Time In Seconds() -> (seconds since 1Jan1904=w52:timestamp)
        n35 = feedback-in #5(w52) -> ()
        n36 = feedback #5(w52) -> (w53:timestamp)
        n37 = call "oldVisionToGame.vi"("VSSRef"=w42, "Defense stretch"="Defense\n stretch", "Team/ Side"=w59, "Defense width"="Defense\n width", "error in (no error)"=w80, "touch"=w49, "IA State"=w56, "Game in"=w69) -> ("Game out"=w44:refnum<class "Game.lvclass">)  [unwired: 2 in, 1 out]
        n38 = Subtract(x=w52, y=w53) -> (x-y=w51:dbl)
        n39 = local read "tempo udp"() -> (w50:dbl)
        n40 = property class="Game" props=["Referee"](reference=w44) -> ()  [unwired: 1 in, 3 out]
        n41 = call "SetVisionFPS.vi"("tempo UDP"=w50, "tempo Vision"=w51, "Vision in"=w55) -> ()  [unwired: 6 in, 3 out]
        n42 = Divide(x=1000.0, y=80.0) -> (x/y=w46:dbl)
        n43 = Wait (ms)(milliseconds to wait=w46) -> ()  [unwired: 1 out]
      }
      frame #1 {
        n44 = in-place {
          in-place-border: w89 -> [w93]
          n45 = in-place-dvr #6(w90) -> (w94:refnum<class "Game.lvclass">)  [unwired: 1 out]
          n46 = call "BundleAll.vi"("Game in\natualized"=w93, "Game in"=w94) -> ("Game out"=w92:refnum<class "Game.lvclass">)  [unwired: 8 in, 1 out]
          n47 = in-place-dvr #6(w92) -> ()  [unwired: 2 out]
        }
        n48 = in-place {
          in-place-border: w87 -> [w91]
          n49 = in-place-dvr #7(w88) -> ()  [unwired: 2 out]
          n50 = in-place-dvr #7(w91) -> ()  [unwired: 2 out]
        }
      }
    }
  }
  n51 = while {
    tunnel: w5 -> [w101]
    tunnel: w11 -> [w96]
    stop <- FALSE stop-if-true
    # "Get Referee Information"
    n52 = flat-sequence {
      tunnel: w101 -> [w109]
      tunnel: [w105] -> w97
      tunnel: w96 -> [w105]
      tunnel: [w104] -> w95
      tunnel: w97 -> [w112]
      tunnel: w95 -> [w111]
      frame #0 {
        # "Get and decode information about\nde referee commands"
        n53 = feedback #8() -> (w102:T36)  [unwired: 1 in]
        n54 = call "filterReferee.vi"("Command"="Command", "Previous Cluster"=w102, "RefBox UDP RX"="RefBox UDP RX", "Vision in"=w109) -> ("SSL Referee Game Status"=w104:T13, "GUI Game Status"=→"GUI Game Status":T13, "Cluster"=w103:T36, "RX"=→"RefBox RX":bool)  [unwired: 2 in, 2 out]
        "SSL Referee Game Status" <- w104
        n55 = feedback-in #8(w103) -> ()
      }
      frame #1 {
        n56 = in-place {
          in-place-border: w111 -> [w113]
          # "Escreve na\nreferência(na memória)\n criada"
          n57 = in-place-dvr #9(w112) -> ()  [unwired: 2 out]
          n58 = in-place-dvr #9(w113) -> ()  [unwired: 2 out]
        }
      }
    }
    n59 = call "FPS Counter.vi"() -> ("Numeric"=→"FPS referee":dbl)  [unwired: 11 in]
    n60 = Wait (ms)(milliseconds to wait=u32 4) -> ()  [unwired: 1 out]
  }
  n61 = while {
    shift-right: [w119] -> _
    shift-left: 0.5 ("New Scale") -> [w126]
    shift-right: [w121] -> _
    shift-left: TRUE ("AutoScale Out") -> [w127]
    tunnel: w5 -> [w125]
    tunnel: w2 -> [w124]
    tunnel: w7 -> [w123]
    stop <- FALSE stop-if-true
    # "Wait necessario\npara 25 FPS"
    # "Draw Field"
    n62 = call "FPS Counter.vi"() -> ("Numeric"=→"FPS Draw Field":dbl)  [unwired: 11 in]
    n63 = feedback #10(0.5 ("New Scale")) -> (w118:dbl)
    n64 = feedback #11(TRUE ("AutoScale Out")) -> (w120:bool)
    n65 = case shown="True" "Draw Field" {
      tunnel: [w128 w139] -> w119
      tunnel: [w129 w138] -> w121
      tunnel: w127 -> [_ w137]
      tunnel: w126 -> [_ w136]
      tunnel: w125 -> [_ w135]
      tunnel: w124 -> [_ w134]
      tunnel: w123 -> [_ w133]
      tunnel: w120 -> [w129 _]
      tunnel: w118 -> [w128 _]
      frame False {
      }
      frame True {
        n66 = flat-sequence {
          tunnel: w137 -> [w148]
          tunnel: w136 -> [w147]
          tunnel: w135 -> [w144]
          tunnel: w134 -> [w143]
          tunnel: w133 -> [w142]
          tunnel: [w150] -> w132
          tunnel: [w149] -> w131
          tunnel: [w140] -> w130
          tunnel: [w162] -> w138
          tunnel: [w163] -> w139
          tunnel: w132 -> [w163]
          tunnel: w131 -> [w162]
          tunnel: w130 -> [w161]
          frame #0 {
            n67 = disable-structure shown="Enabled" {
              disable-tunnel: [w152 1.0 ("Zoom")] -> w146
              frame Enabled {
                n68 = event shown="[0] \"2D Picture\": Mouse Wheel" {
                  selector: _ -> [_ _]
                  dyn-events: _ -> [_ _]
                  timeout: 0 -> [_ _]
                  tunnel: [w153 1.0] -> w152
                  event "2D Picture": Mouse Wheel {
                    n69 = event-data() -> ("Delta"=w157:i32)  [unwired: 1 in]
                    n70 = Greater Than 0?(x=w157) -> (x > 0?=w156:bool)
                    n71 = Select(t=1.2, s=w156, f=0.8) -> (s? t:f=w153:dbl)
                  }
                  event Timeout {
                    n72 = event-data() -> ()  [unwired: 1 in, 3 out]
                  }
                }
              }
              frame Disabled {
              }
            }
            n73 = in-place {
              in-place-border: [w160] -> w141
              n74 = in-place-dvr #12(w142) -> (w160:T19)  [unwired: 1 out]
              n75 = in-place-dvr #12() -> ()  [unwired: 1 in, 2 out]
            }
            n76 = call "drawField.vi"("Vision in"=w144, "AutoScale"=w148, "Game reference"=w143, "Field State Input"=w141, "Scale mm/pixel"=w147, "Draw Targets?"="Draw Targets?", "Zoom"=w146) -> ("AutoScale Out"=w149:bool, "2D Picture"=w140:picture, "Scale Out"=w150:dbl)  [unwired: 4 in, 2 out]
          }
          frame #1 {
            n77 = property on="2D Picture" class="Pict"("Value"=w161) -> ()  [unwired: 2 in, 2 out]
            "2D Picture" <- w161
          }
        }
      }
    }
    n78 = feedback-in #10(w119) -> ()
    n79 = feedback-in #11(w121) -> ()
  }
  n80 = disable-structure shown="Enabled" {
    frame Disabled {
      n81 = while {
        stop <- FALSE stop-if-true
        n82 = event shown="[0] \"2D Picture\": Mouse Wheel" {
          selector: _ -> [_ _]
          dyn-events: _ -> [_ _]
          timeout: 0 -> [_ _]
          tunnel: [w169 1.0] -> w166
          event "2D Picture": Mouse Wheel {
            n83 = event-data() -> ("Delta"=w173:i32)  [unwired: 1 in]
            n84 = Greater Than 0?(x=w173) -> (x > 0?=w172:bool)
            n85 = Select(t=1.2, s=w172, f=0.8) -> (s? t:f=w169:dbl)
          }
          event Timeout {
            n86 = event-data() -> ()  [unwired: 1 in, 3 out]
          }
        }
        "zoom" <- w166
        n87 = call "FPS Counter.vi"() -> ("Numeric"=→"FPS Mouse":dbl)  [unwired: 11 in]
        n88 = Wait (ms)(milliseconds to wait=u32 10) -> ()  [unwired: 1 out]
      }
    }
    frame Enabled {
      n89 = while {
        stop <- FALSE stop-if-true
        # "Wait necessario\npara 25 FPS"
        n90 = call "FPS Counter.vi"() -> ("Numeric"=→"FPS Print Field":dbl)  [unwired: 11 in]
        n91 = Wait (ms)(milliseconds to wait=u32 30) -> ()  [unwired: 1 out]
        n92 = property on="2D Picture" class="Pict" props=["Value"]() -> ()  [unwired: 2 in, 3 out]
      }
    }
  }
  n93 = disable-structure shown="Enabled" {
    disable-tunnel: w2 -> [w178 _]
    frame Enabled {
      n94 = while {
        tunnel: w178 -> [w186]
        stop <- FALSE stop-if-true
        n95 = disable-structure shown="Enabled" {
          frame Disabled {
            n96 = local read "FPS vision"() -> (w192:dbl)
            n97 = Bundle("FPS vision"=w192) -> (w191:cluster{"FPS vision":dbl})  [unwired: 1 in]
            n98 = local read "FPS Navigation"() -> (w189:dbl)
            n99 = local read "FPS Offensive"() -> (w190:dbl)
            n100 = local read "FPS Com"() -> (w188:dbl)
            n101 = Bundle("FPS Navigation"=w189) -> ()  [unwired: 1 in, 1 out]
            n102 = Bundle("FPS Com"=w188) -> ()  [unwired: 1 in, 1 out]
            n103 = Bundle("FPS Offensive"=w190) -> ()  [unwired: 1 in, 1 out]
          }
          frame Enabled {
          }
        }
        n104 = call "FPS Counter.vi"() -> ("Numeric"=→"FPS Graph":dbl)  [unwired: 11 in]
        n105 = in-place {
          in-place-border: [w193] -> w179
          n106 = in-place-dvr #13(w186) -> (w193:refnum<class "Game.lvclass">)  [unwired: 1 out]
          n107 = in-place-dvr #13() -> ()  [unwired: 1 in, 2 out]
        }
        n108 = Wait (ms)(milliseconds to wait=u32 45) -> ()  [unwired: 1 out]
        n109 = case shown="True" "Draw Graphs" {
          tunnel: w179 -> [_ w201]
          tunnel: "id 1" -> [_ w196]
          tunnel: "id 2" -> [_ w195]
          tunnel: "id 3" -> [_ w194]
          frame False {
          }
          frame True {
            n110 = call-dynamic "PlotGraphs.vi"("Game in"=w201, "id 1"=w196, "id 2"=w195, "id 3"=w194) -> ("ball"=→"ball":dbl, "Robot 1"=→"Robot":cluster{"Modulo":dbl, "Modulo":dbl}, "Robot 2"=→"Robot":cluster{"Modulo":dbl, "Modulo":dbl}, "Robot 3"=→"Robot":cluster{"Modulo":dbl, "Modulo":dbl})  [unwired: 6 in, 2 out]
          }
        }
      }
    }
    frame Disabled {
    }
  }
  n111 = while {
    tunnel: w2 -> [w211]
    stop <- FALSE stop-if-true
    # "Keeper"
    n112 = flat-sequence {
      tunnel: w211 -> [w225]
      tunnel: [w224] -> w210
      tunnel: [w223] -> w209
      tunnel: [w222] -> w208
      tunnel: w203 -> [w215]
      tunnel: w202 -> [w214]
      tunnel: [w250] -> _
      tunnel: w210 -> [w250]
      tunnel: w209 -> [w249]
      tunnel: w208 -> [w248]
      frame #0 {
        w216 = 40.0
        n113 = in-place {
          in-place-border: [w247] -> w220
          n114 = in-place-dvr #14(w225) -> (w247:refnum<class "Game.lvclass">)  [unwired: 1 out]
          n115 = in-place-dvr #14() -> (w224:refnum<data-value>)  [unwired: 1 in, 1 out]
        }
        n116 = local read "Project"() -> (w219:T4)
        n117 = Greater Or Equal?(x=w215, y=w216) -> (x >= y?=w217:bool)
        n118 = Less Or Equal?(x=w214, y=w216) -> (x <= y?=w218:bool)
        n119 = And(x=w217, y=w218) -> (x .and. y?=w213:bool)
        n120 = case shown="\"VSS\"" w219 {
          tunnel: [w227 w242] -> w221
          tunnel: w220 -> [w226 w246]
          tunnel: w213 -> [_ w234]
          frame "SSL", Default {
            n121 = call "chooseKeeperPlay.vi"("Game in"=w226) -> ("error out"=w232:errorcluster, "Game out"=w228:refnum<class "Game.lvclass">)  [unwired: 9 in]
            n122 = call-dynamic "pickKeeperRobots.vi"("error in (no error)"=w232, "Game in"=w228) -> ("error out"=w233:errorcluster, "Game out"=w230:refnum<class "Game.lvclass">)  [unwired: 8 in]
            n123 = call-dynamic "executeKeeperPlay.vi"("error in (no error)"=w233, "Game in"=w230) -> ("error out"=w231:errorcluster, "Game out"=w229:refnum<class "Game.lvclass">)  [unwired: 8 in]
            n124 = call-dynamic "pathPlanningKeeper.vi"("error in (no error)"=w231, "Game in"=w229) -> ("Game out"=w227:refnum<class "Game.lvclass">)  [unwired: 8 in, 1 out]
          }
          frame "VSS" {
            w236 = T37."Stop" ("VssPlay")
            n125 = Build Array(w236, w236, w236) -> (w235:T38)
            n126 = feedback #15(w235) -> (w237:T38)
            n127 = call-dynamic "choosePlayVSS.vi"("queue"=w237, "Game in"=w246) -> ("error out"=w241:errorcluster, "output queue"=w238:T38, "Game out"=w245:refnum<class "Game.lvclass">)  [unwired: 7 in]
            n128 = feedback-in #15(w238) -> ()
            n129 = call-dynamic "pickRobotsVSS.vi"("error in (no error)"=w241, "Game in"=w245) -> ("error out"=w240:errorcluster, "Game out"=w244:refnum<class "Game.lvclass">)  [unwired: 8 in]
            n130 = call-dynamic "executePlayVSS.vi"("error in (no error)"=w240, "Game in"=w244) -> ("error out"=w239:errorcluster, "Game out"=w243:refnum<class "Game.lvclass">)  [unwired: 8 in]
            n131 = call "pathPlanningVSS.vi"("error in (no error) 2"=w239, "Line?"=w234, "Game in 2"=w243) -> ("Game out 2"=w242:refnum<class "Game.lvclass">)  [unwired: 7 in, 1 out]
          }
        }
        n132 = property class="Game"(reference=w221) -> ("KeeperTeam"=w223:refnum<class "Ally.lvclass">, "Playbook"=w222:refnum<class "Playbook.lvclass">)  [unwired: 1 in, 2 out]
      }
      frame #1 {
        n133 = in-place {
          in-place-border: w249 -> [w252]
          in-place-border: w248 -> [w253]
          n134 = in-place-dvr #16(w250) -> (w251:refnum<class "Game.lvclass">)  [unwired: 1 out]
          n135 = property class="Game"(reference=w251, "KeeperTeam"=w252, "Playbook"=w253) -> (reference out=w254:refnum<class "Game.lvclass">)  [unwired: 1 in, 1 out]
          n136 = in-place-dvr #16(w254) -> ()  [unwired: 2 out]
        }
      }
    }
    n137 = local read "FPS vision"() -> (w203:dbl)
    n138 = Subtract(x=w203, y=2.0) -> (x-y=w204:dbl)
    n139 = Divide(x=1000.0, y=w204) -> (x/y=w207:dbl)
    n140 = Wait (ms)(milliseconds to wait=w207) -> ()  [unwired: 1 out]
    n141 = call "FPS Counter.vi"() -> ("Numeric"=w202:dbl)  [unwired: 11 in]
    "FPS Keeper" <- w202
  }
  n142 = while {
    tunnel: w2 -> [w264]
    stop <- FALSE stop-if-true
    # "Event Generator"
    n143 = local read "FPS vision"() -> (w257:dbl)
    n144 = flat-sequence {
      tunnel: w264 -> [w270]
      tunnel: [w267] -> w263
      tunnel: [w266] -> w262
      tunnel: w263 -> [w273]
      tunnel: w262 -> [w272]
      frame #0 {
        n145 = in-place {
          in-place-border: [w271] -> w269
          n146 = in-place-dvr #17(w270) -> (w271:refnum<class "Game.lvclass">)  [unwired: 1 out]
          n147 = in-place-dvr #17() -> (w267:refnum<data-value>)  [unwired: 1 in, 1 out]
        }
        n148 = call-dynamic "Generate_events.vi"("Game in"=w269, "Events in"=refnum<class "Events.lvclass"> refnum) -> ("touch"=→"touch":bool, "Events out"=w266:refnum<class "Events.lvclass">)  [unwired: 7 in, 1 out]
      }
      frame #1 {
        n149 = in-place {
          in-place-border: w272 -> [w275]
          n150 = in-place-dvr #18(w273) -> (w276:refnum<class "Game.lvclass">)  [unwired: 1 out]
          n151 = property class="Game"(reference=w276, "EventsRef"=w275) -> (reference out=w274:refnum<class "Game.lvclass">)  [unwired: 1 in, 1 out]
          n152 = in-place-dvr #18(w274) -> ()  [unwired: 2 out]
        }
      }
    }
    n153 = Subtract(x=w257, y=2.0) -> (x-y=w255:dbl)
    n154 = call "FPS Counter.vi"() -> ("Numeric"=→"FPS Events":dbl)  [unwired: 11 in]
    n155 = Divide(x=1000.0, y=w255) -> (x/y=w258:dbl)
    n156 = Wait (ms)(milliseconds to wait=w258) -> ()  [unwired: 1 out]
  }
  n157 = while {
    tunnel: w2 -> [w289]
    stop <- w277 stop-if-true
    # "dont execute \"while\" with vss code"
    # "Defensive"
    n158 = flat-sequence {
      tunnel: w289 -> [w301]
      tunnel: [w293] -> w288
      tunnel: [w292] -> w287
      tunnel: [w291] -> w286
      tunnel: w288 -> [w304]
      tunnel: w287 -> [w303]
      tunnel: w286 -> [w305]
      frame #0 {
        n159 = in-place {
          in-place-border: [w302] -> w294
          n160 = in-place-dvr #19(w301) -> (w302:refnum<class "Game.lvclass">)  [unwired: 1 out]
          n161 = in-place-dvr #19() -> (w291:refnum<data-value>)  [unwired: 1 in, 1 out]
        }
        n162 = call-dynamic "chooseDefensivePlay.vi"("Game in"=w294) -> ("error out"=w299:errorcluster, "Game out"=w300:refnum<class "Game.lvclass">)  [unwired: 9 in]
        n163 = call-dynamic "pickDefensiveRobots.vi"("error in (no error)"=w299, "Game in"=w300) -> ("error out"=w297:errorcluster, "Game out"=w298:refnum<class "Game.lvclass">)  [unwired: 8 in]
        n164 = call-dynamic "executeDefensivePlay.vi"("error in (no error)"=w297, "Game in"=w298) -> ("error out"=w296:errorcluster, "Game out"=w295:refnum<class "Game.lvclass">)  [unwired: 8 in]
        n165 = call-dynamic "pathPlanningDefensive.vi"("error in (no error)"=w296, "Game in"=w295) -> ("Game out"=w290:refnum<class "Game.lvclass">)  [unwired: 8 in, 1 out]
        n166 = property class="Game"(reference=w290) -> ("DefensiveTeam"=w293:refnum<class "Ally.lvclass">, "Playbook"=w292:refnum<class "Playbook.lvclass">)  [unwired: 1 in, 2 out]
      }
      frame #1 {
        n167 = in-place {
          in-place-border: w304 -> [w307]
          in-place-border: w303 -> [w308]
          n168 = in-place-dvr #20(w305) -> (w306:refnum<class "Game.lvclass">)  [unwired: 1 out]
          n169 = property class="Game"(reference=w306, "DefensiveTeam"=w307, "Playbook"=w308) -> (reference out=w309:refnum<class "Game.lvclass">)  [unwired: 1 in, 1 out]
          n170 = in-place-dvr #20(w309) -> ()  [unwired: 2 out]
        }
      }
    }
    n171 = local read "FPS vision"() -> (w282:dbl)
    n172 = Subtract(x=w282, y=2.0) -> (x-y=w280:dbl)
    n173 = Divide(x=1000.0, y=w280) -> (x/y=w284:dbl)
    n174 = Wait (ms)(milliseconds to wait=w284) -> ()  [unwired: 1 out]
    n175 = local read "Project"() -> (w278:T4)
    n176 = Equal?(x=w278, y=Project."VSS" ("Project 2")) -> (x = y?=w277:bool)
    n177 = call "FPS Counter.vi"() -> ("Numeric"=→"FPS Defensive":dbl)  [unwired: 11 in]
  }
  n178 = while {
    tunnel: w2 -> [w322]
    stop <- w310 stop-if-true
    # "dont execute \"while\" with vss code"
    # "Offensive"
    n179 = local read "FPS vision"() -> (w313:dbl)
    n180 = flat-sequence {
      tunnel: w322 -> [w340]
      tunnel: [w334] -> w319
      tunnel: [w333] -> w318
      tunnel: [w332] -> w317
      tunnel: w314 -> [w330]
      tunnel: w313 -> [w327]
      tunnel: w319 -> [w344]
      tunnel: w318 -> [w343]
      tunnel: w317 -> [w342]
      frame #0 {
        w326 = 40.0
        # "Pass unique line"
        n181 = in-place {
          in-place-border: [w341] -> w323
          n182 = in-place-dvr #21(w340) -> (w341:refnum<class "Game.lvclass">)  [unwired: 1 out]
          n183 = in-place-dvr #21() -> (w332:refnum<data-value>)  [unwired: 1 in, 1 out]
        }
        n184 = call-dynamic "chooseOffensivePlay.vi"("Game in"=w323) -> ("error out"=w337:errorcluster, "Game out"=w336:refnum<class "Game.lvclass">)  [unwired: 9 in]
        n185 = call-dynamic "pickOffensiveRobots.vi"("error in (no error)"=w337, "Game in"=w336) -> ("error out"=w338:errorcluster, "Game out"=w335:refnum<class "Game.lvclass">)  [unwired: 8 in]
        n186 = call-dynamic "executeOffensivePlay.vi"("error in (no error)"=w338, "Game in"=w335) -> ("error out"=w339:errorcluster, "Game out"=w324:refnum<class "Game.lvclass">)  [unwired: 8 in]
        n187 = Greater Or Equal?(x=w327, y=w326) -> (x >= y?=w328:bool)
        n188 = Less Or Equal?(x=w330, y=w326) -> (x <= y?=w329:bool)
        n189 = And(x=w328, y=w329) -> (x .and. y?=w325:bool)
        n190 = call-dynamic "pathPlanningOffensive.vi"("error in (no error)"=w339, "Line?"=w325, "Game in"=w324) -> ("Game out"=w331:refnum<class "Game.lvclass">)  [unwired: 7 in, 1 out]
        n191 = property class="Game"(reference=w331) -> ("OffensiveTeam"=w334:refnum<class "Ally.lvclass">, "Playbook"=w333:refnum<class "Playbook.lvclass">)  [unwired: 1 in, 2 out]
      }
      frame #1 {
        n192 = in-place {
          in-place-border: w344 -> [w348]
          in-place-border: w343 -> [w347]
          n193 = in-place-dvr #22(w342) -> (w345:refnum<class "Game.lvclass">)  [unwired: 1 out]
          n194 = property class="Game"(reference=w345, "OffensiveTeam"=w348, "Playbook"=w347) -> (reference out=w346:refnum<class "Game.lvclass">)  [unwired: 1 in, 1 out]
          n195 = in-place-dvr #22(w346) -> ()  [unwired: 2 out]
        }
      }
    }
    n196 = Subtract(x=w313, y=2.0) -> (x-y=w316:dbl)
    n197 = Divide(x=1000.0, y=w316) -> (x/y=w320:dbl)
    n198 = Wait (ms)(milliseconds to wait=w320) -> ()  [unwired: 1 out]
    n199 = call "FPS Counter.vi"() -> ("Numeric"=w314:dbl)  [unwired: 11 in]
    "FPS Offensive" <- w314
    n200 = local read "Project"() -> (w312:T4)
    n201 = Equal?(x=w312, y=Project."VSS" ("Project 2")) -> (x = y?=w310:bool)
  }
  n202 = while {
    tunnel: w2 -> [w367]
    stop <- FALSE stop-if-true
    # "Set Parameters"
    n203 = flat-sequence {
      tunnel: w367 -> [w372]
      tunnel: [w372] -> w365
      tunnel: ["Offensive ids"] -> w364
      tunnel: ["Defensive ids"] -> w363
      tunnel: ["zigzag Points"] -> w362
      tunnel: ["TestMode IDS"] -> w361
      tunnel: ["TestMode"] -> w360
      tunnel: ["Tests"] -> w359
      tunnel: ["Test"] -> w358
      tunnel: ["AI Parameters"] -> w357
      tunnel: ["AttakingOurselves"] -> w356
      tunnel: ["Debug"] -> w355
      tunnel: ["ChipKick activated"] -> w354
      tunnel: ["PID gains Vel D"] -> w353
      tunnel: ["PID gains Angle"] -> w352
      tunnel: ["Project"] -> w350
      tunnel: ["AI Parameters VSS"] -> w349
      tunnel: w365 -> [w398]
      tunnel: w364 -> [w400]
      tunnel: w363 -> [w399]
      tunnel: w362 -> [w397]
      tunnel: w361 -> [w396]
      tunnel: w360 -> [w395]
      tunnel: w359 -> [w394]
      tunnel: w358 -> [w393]
      tunnel: w357 -> [w392]
      tunnel: w356 -> [w391]
      tunnel: w355 -> [w390]
      tunnel: w354 -> [w389]
      tunnel: w353 -> [w388]
      tunnel: w352 -> [w387]
      tunnel: w350 -> [w386]
      tunnel: w349 -> [w385]
      frame #0 {
        n204 = local write "Project"("Project") -> ()
      }
      frame #1 {
        n205 = in-place {
          in-place-border: w400 -> [w467]
          in-place-border: w399 -> [w466]
          in-place-border: w397 -> [w415]
          in-place-border: w396 -> [w461]
          in-place-border: w395 -> [w460]
          in-place-border: w394 -> [w459]
          in-place-border: w393 -> [w457]
          in-place-border: w392 -> [w456]
          in-place-border: w391 -> [w423]
          in-place-border: w390 -> [w420]
          in-place-border: w389 -> [w422]
          in-place-border: w388 -> [w418]
          in-place-border: w387 -> [w417]
          in-place-border: w386 -> [w403]
          in-place-border: w385 -> [w402]
          n206 = in-place-dvr #23(w398) -> (w468:refnum<class "Game.lvclass">)  [unwired: 1 out]
          n207 = property class="Game"(reference=w468, "Offensive ids"=w467, "Defensive ids"=w466, "Test"=w457, "TestMode IDs"=w461, "TestMode"=w460, "Tests"=w459) -> (reference out=w464:refnum<class "Game.lvclass">, "Parameters.lvclass"=w465:refnum<class "Parameters.lvclass">)  [unwired: 1 in, 1 out]
          n208 = Unbundle By Name(w456) -> ("Area"=w455:enum16{"Circular", "Square"}, "DistanceBehindAttacker"=w454:dbl, "DistanceInFrontOfAttacker"=w453:dbl, "DistanceStop"=w452:dbl, "DistanceToBallOut"=w451:dbl, "DistanceToGoAroundBall"=w450:dbl, "DistanceToGoAroundBallPass"=w449:dbl, "DistanceToKickingAngle"=w424:dbl, "Force++"=w425:dbl, "KickAngle"=w426:dbl, "KickEps"=w427:dbl, "KickForce"=w428:dbl, "KickRange"=w429:dbl, "MaxAcceleration"=w430:dbl, "MaxControlIncrement"=w431:dbl, "MaxDeceleration"=w432:dbl, "MaxOutputAngle"=w433:dbl, "MaxOutputXY"=w434:dbl, "MinDistToKick"=w435:dbl, "PassAngle"=w436:dbl, "Type of Defense"=w437:enum16{"Barreira", "Manmark"}, "Type of Marker"=w438:enum16{"BlockEnemyPass", "BlockOurGoal"}, "AttackerFarback"=w439:dbl, "TouchDist"=w440:dbl, "TimeoutDistanceInY"=w441:dbl, "TimeoutDistanceInX"=w442:dbl, "TimeoutDistanceBetweenRobots"=w443:dbl, "MaxVelBallToBeginDuelist"=w444:dbl, "DistForPossession"=w445:dbl, "DistanceForStealBall"=w446:dbl, "Defensive Marker"=w447:enum16{"SecondMostDangerous", "MostDangerous"}, "AngularToleranceForPossession"=w448:dbl, "ZigZagAngle"=w421:dbl, "PID gains Vel"=w419:T39, "Number of Offensive"=w416:T40, "Shoot Out?"=w414:bool, "DefenseAvoidArea"=w413:bool, "InvertKick"=w412:dbl[], "shootOutForce"=w411:dbl, "dtPosEst\nBall"=w410:dbl, "AttackerIgnoreBallObstacle"=w409:dbl, "BarrierDistanceToArea"=w408:dbl, "SimplePass"=w407:bool, "GoalieInFront\nGoal"=w406:dbl, "RollToPass"=w405:bool, "VelNearBall"=w404:dbl, "OldRRT"=w401:bool)  [unwired: 2 out]
          n209 = property class="Parameters.lvclass"(reference=w465, "Area"=w455, "DistanceBehindAttacker"=w454, "DistanceInFrontOfAttacker"=w453, "DistanceStop"=w452, "DistanceToBallOut"=w451, "DistanceToGoAroundBall"=w450, "DistanceToGoAroundBallPass"=w449, "DistanceToKickingAngle"=w424, "Force++"=w425, "KickAngle"=w426, "KickEps"=w427, "KickForce"=w428, "KickRange"=w429, "MaxAcceleration"=w430, "MaxControlIncrement"=w431, "MaxDeceleration"=w432, "MaxOutputAngle"=w433, "MaxOutputXY"=w434, "MinDistToKick"=w435, "PassAngle"=w436, "Type of Defense"=w437, "Type of Marker"=w438, "AttackerFarback"=w439, "TouchDistance"=w440, "TimeoutDistanceInY"=w441, "TimeoutDistanceInX"=w442, "TimeoutDistanceBetweenRobots"=w443, "MaxVelBallToBeginDuelist"=w444, "DistanceForPossession"=w445, "DistanceForaStillBall"=w446, "Defensive Marker"=w447, "AngularToleranceForPossession"=w448, "zigzag Points"=w415, "AttakingOurselves"=w423, "Debug"=w420, "ChipKick activated"=w422, "Angle"=w421, "PID gains Vel"=w419, "PID gains Vel_desired"=w418, "PID gains Angle"=w417, "Number of Offesnive"=w416, "Shoot Out_"=w414, "DefenseAvoidArea"=w413, "InvertKick"=w412, "ShootOutForce"=w411, "dtPosEstBall"=w410, "AttackerIgnoreBallObstacle"=w409, "BarrierDistanceToArea"=w408, "SimplePass"=w407, "GoalieInFrontGoal"=w406, "RollToPass"=w405, "VelNearBall"=w404, "Project"=w403, "VSSParams"=w402, "OldRRT"=w401) -> (reference out=w462:refnum<class "Parameters.lvclass">, error out=→"error out":errorcluster)  [unwired: 1 in]
          n210 = property class="Game"(reference=w464, "Parameters.lvclass"=w462) -> (reference out=w463:refnum<class "Game.lvclass">)  [unwired: 1 in, 1 out]
          n211 = in-place-dvr #23(w463) -> ()  [unwired: 2 out]
        }
      }
    }
    n212 = call "FPS Counter.vi"() -> ("Numeric"=→"FPS SetParameters":dbl)  [unwired: 11 in]
    n213 = Wait (ms)(milliseconds to wait=u32 30) -> ()  [unwired: 1 out]
  }
  n214 = while {
    tunnel: w2 -> [w472]
    stop <- FALSE stop-if-true
    # "Navigation"
    n215 = flat-sequence {
      tunnel: [w493] -> w476
      tunnel: w472 -> [w490]
      tunnel: [w480] -> w471
      tunnel: [w478] -> w470
      tunnel: [w507] -> _
      tunnel: w476 -> [w507]
      tunnel: w471 -> [w506]
      tunnel: w470 -> [w505]
      frame #0 {
        n216 = in-place {
          in-place-border: [w504] -> w494
          n217 = in-place-dvr #24(w490) -> (w504:refnum<class "Game.lvclass">)  [unwired: 1 out]
          n218 = in-place-dvr #24() -> (w493:refnum<data-value>)  [unwired: 1 in, 1 out]
        }
        n219 = call-dynamic "NavigationOffensive.vi"("Game in"=w494) -> ("Game out"=w492:refnum<class "Game.lvclass">)  [unwired: 9 in, 1 out]
        n220 = call-dynamic "NavigationDefensive.vi"("Game in"=w494) -> ("Game out"=w491:refnum<class "Game.lvclass">)  [unwired: 9 in, 1 out]
        n221 = call-dynamic "NavigationKeeper.vi"("Game in"=w494) -> ("Game out"=w479:refnum<class "Game.lvclass">)  [unwired: 9 in, 1 out]
        n222 = property class="Game"(reference=w491) -> ("DefensiveTeam"=w481:refnum<class "Ally.lvclass">)  [unwired: 1 in, 2 out]
        n223 = property class="Game"(reference=w492) -> ("OffensiveTeam"=w482:refnum<class "Ally.lvclass">)  [unwired: 1 in, 2 out]
        n224 = property class="Game"(reference=w479) -> ("AllyRef"=w478:refnum<class "Ally.lvclass">)  [unwired: 1 in, 2 out]
        n225 = property class="Game"(reference=w479) -> ("KeeperTeam"=w483:refnum<class "Ally.lvclass">)  [unwired: 1 in, 2 out]
        n226 = property class="Ally"(reference=w481) -> ("RobotRef"=w484:refnum<class "Robot.lvclass">[])  [unwired: 1 in, 2 out]
        n227 = property class="Ally"(reference=w483) -> ("RobotRef"=w489:refnum<class "Robot.lvclass">[])  [unwired: 1 in, 2 out]
        n228 = property class="Ally"(reference=w482) -> ("RobotRef"=w486:refnum<class "Robot.lvclass">[])  [unwired: 1 in, 2 out]
        n229 = for {
          tunnel: w489 -> [w503] mode=indexing
          shift-right: [w501] -> w487
          shift-left: refnum<class "Robot.lvclass">[] [] -> [w502]
          n230 = Insert Into Array(array=w502, new element=w503) -> (w501:refnum<class "Robot.lvclass">[])  [unwired: 1 in]
        }
        n231 = for {
          tunnel: w486 -> [w500] mode=indexing
          shift-right: [w498] -> w485
          shift-left: w487 -> [w499]
          n232 = Insert Into Array(array=w499, new element=w500) -> (w498:refnum<class "Robot.lvclass">[])  [unwired: 1 in]
        }
        n233 = for {
          tunnel: w484 -> [w497] mode=indexing
          shift-right: [w495] -> w480
          shift-left: w485 -> [w496]
          n234 = Insert Into Array(array=w496, new element=w497) -> (w495:refnum<class "Robot.lvclass">[])  [unwired: 1 in]
        }
      }
      frame #1 {
        n235 = in-place {
          in-place-border: w506 -> [w509]
          in-place-border: w505 -> [w508]
          n236 = in-place-dvr #25(w507) -> (w511:refnum<class "Game.lvclass">)  [unwired: 1 out]
          n237 = property class="Ally"(reference=w508, "RobotRef"=w509) -> (reference out=w510:refnum<class "Ally.lvclass">)  [unwired: 1 in, 1 out]
          n238 = property class="Game"(reference=w511, "NavigationTeam"=w510) -> (reference out=w512:refnum<class "Game.lvclass">)  [unwired: 1 in, 1 out]
          n239 = in-place-dvr #25(w512) -> ()  [unwired: 2 out]
        }
      }
    }
    n240 = call "FPS Counter.vi"() -> ("Numeric"=→"FPS Navigation":dbl)  [unwired: 11 in]
    n241 = Divide(x=1000.0, y=70.0) -> (x/y=w475:dbl)
    n242 = Wait (ms)(milliseconds to wait=w475) -> ()  [unwired: 1 out]
  }
  n243 = while "VSS Ref Placement" {
    tunnel: w2 -> [w523]
    stop <- FALSE stop-if-true
    n244 = in-place {
      in-place-border: [w524] -> w519
      n245 = in-place-dvr #26(w523) -> (w524:refnum<class "Game.lvclass">)  [unwired: 1 out]
      n246 = in-place-dvr #26() -> ()  [unwired: 1 in, 2 out]
    }
    n247 = call "communicateVSSRefPlacement.vi"("SEND?"="SEND?", "VSSRef Replacement infos"="VSSRef Replacement infos", "Game"=w519, "Communication in"=refnum<class "Communication.lvclass"> refnum) -> ()  [unwired: 6 in, 2 out]
    n248 = local read "FPS vision"() -> (w515:dbl)
    n249 = Subtract(x=w515, y=5.0) -> (x-y=w518:dbl)
    n250 = Divide(x=1000.0, y=w518) -> (x/y=w514:dbl)
    n251 = Wait (ms)(milliseconds to wait=w514) -> ()  [unwired: 1 out]
  }
  n252 = while {
    tunnel: w2 -> [w554]
    stop <- FALSE stop-if-true
    n253 = local read "FPS vision"() -> (w532:dbl)
    n254 = Subtract(x=w532, y=5.0) -> (x-y=w529:dbl)
    n255 = in-place {
      in-place-border: [w574] -> w527
      n256 = in-place-dvr #27(w554) -> (w574:refnum<class "Game.lvclass">)  [unwired: 1 out]
      n257 = in-place-dvr #27() -> (w549:refnum<data-value>)  [unwired: 1 in, 1 out]
    }
    n258 = Divide(x=1000.0, y=w529) -> (x/y=w533:dbl)
    n259 = local read "FIRASim?"() -> (w525:bool)
    n260 = Wait (ms)(milliseconds to wait=w533) -> ()  [unwired: 1 out]
    n261 = call-dynamic "communicate.vi"("Communication in"="Communication in", "Game"=w527, "Com UDP"="Com UDP", "Com Serial"="Com Serial", "Com SOS"="Com SOS", "FIRASim?"=w525) -> ("Comm TX FPS"=→"FPS Com":dbl, "AllyRef"=w550:refnum<class "Ally.lvclass">)  [unwired: 6 in, 2 out]
    n262 = disable-structure shown="Disabled" {
      disable-tunnel: w550 -> [w556 _]
      disable-tunnel: w549 -> [w555 _]
      frame Disabled {
        n263 = in-place {
          in-place-border: w556 -> [w557]
          n264 = in-place-dvr #28(w555) -> (w558:refnum<class "Game.lvclass">)  [unwired: 1 out]
          n265 = property class="Game"(reference=w558, "AllyRef"=w557) -> ()  [unwired: 1 in, 2 out]
          n266 = in-place-dvr #28() -> ()  [unwired: 1 in, 2 out]
        }
      }
      frame Enabled {
      }
    }
    n267 = property class="Game"(reference=w549) -> ("Referee"=w539:refnum<class "Referee.lvclass">, "KeeperTeam"=w548:refnum<class "Ally.lvclass">, "OffensiveTeam"=w547:refnum<class "Ally.lvclass">, "DefensiveTeam"=w546:refnum<class "Ally.lvclass">)  [unwired: 1 in, 2 out]
    n268 = property class="Ally"(reference=w546) -> ("RobotRef"=w543:refnum<class "Robot.lvclass">[], "DefensivePlay"=→"DefensivePlay":T12)  [unwired: 1 in, 2 out]
    n269 = property class="Ally"(reference=w547) -> ("RobotRef"=w544:refnum<class "Robot.lvclass">[], "OffensivePlay"=→"OffensivePlay":T9)  [unwired: 1 in, 2 out]
    n270 = property class="Ally"(reference=w548) -> ("RobotRef"=w545:refnum<class "Robot.lvclass">[], "KeeperPlay"=→"KeeperPlay":T8)  [unwired: 1 in, 2 out]
    n271 = property class="Referee"(reference=w539) -> ("command_interpreted"=→"command_interpreted":T14)  [unwired: 1 in, 2 out]
    n272 = for {
      tunnel: w544 -> [w568] mode=indexing
      tunnel: [w565] -> w536 mode=indexing
      n273 = property class="Robot"(reference=w568) -> ("id"=w567:i32, "role"=w566:T10, "tactic"=w564:T11)  [unwired: 1 in, 2 out]
      n274 = Bundle("id"=w567, "role"=w566, "tactic"=w564) -> (w565:cluster{"id":i32, "role":T10, "tactic":T11})  [unwired: 1 in]
    }
    "Offensive Team" <- w536
    n275 = for {
      tunnel: w545 -> [w573] mode=indexing
      tunnel: [w570] -> w537 mode=indexing
      n276 = property class="Robot"(reference=w573) -> ("id"=w572:i32, "role"=w571:T10, "tactic"=w569:T11)  [unwired: 1 in, 2 out]
      n277 = Bundle("id"=w572, "role"=w571, "tactic"=w569) -> (w570:cluster{"id":i32, "role":T10, "tactic":T11})  [unwired: 1 in]
    }
    "Keeper Team" <- w537
    n278 = for {
      tunnel: w543 -> [w563] mode=indexing
      tunnel: [w560] -> w535 mode=indexing
      n279 = property class="Robot"(reference=w563) -> ("id"=w562:i32, "role"=w561:T10, "tactic"=w559:T11)  [unwired: 1 in, 2 out]
      n280 = Bundle("id"=w562, "role"=w561, "tactic"=w559) -> (w560:cluster{"id":i32, "role":T10, "tactic":T11})  [unwired: 1 in]
    }
    "Defensive Team" <- w535
  }
  "Exit" <- 0 ("Exit")
